vi "MSScript_Format_UpdDO.vi"(9 "ValueArray":string[](array[string]), 10 "TagArray":string[](array[string]), 11 "MSScript.lvclass":refnum<class "MSScript.lvclass">) -> (0 "ValueErrorArray":bool[](array[boolean]), 1 "TagErrorArray":bool[](array[boolean]), 2 "ParamErrorArray":bool[](array[boolean]), 3 "Data":variant, 4 "#ofParamError":bool)   [LabVIEW 2018, in "MSScript.lvclass"]
uses:
  MSScript.lvclass
  Ctl/MSEditorParam updDO.ctl
  MSScript_Transform_UIntArray.vi
  MSScript_Transform_BooleanArray.vi
panel:
  in  "ParamValueOutput":T1={"func"=[1, 2, 0, 0], "val"=[FALSE, FALSE, FALSE, FALSE]}
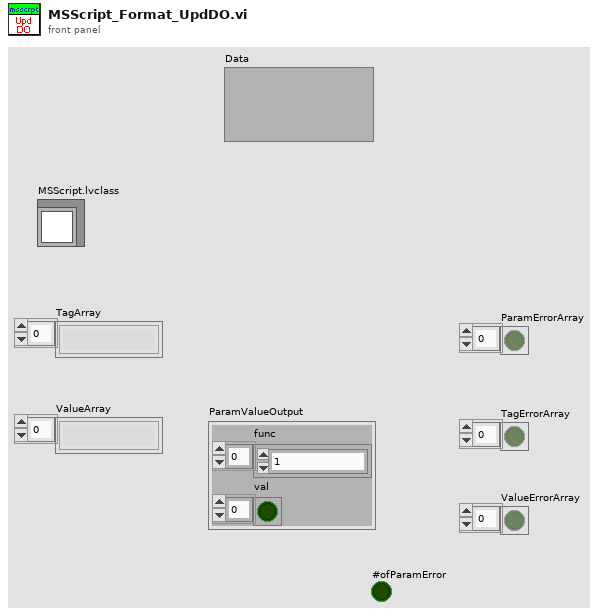
[diagram p1: front panel]
types:
  T1 = typedef "MSEditorParam updDO.ctl" = cluster{"func":u32[], "val":bool[]}
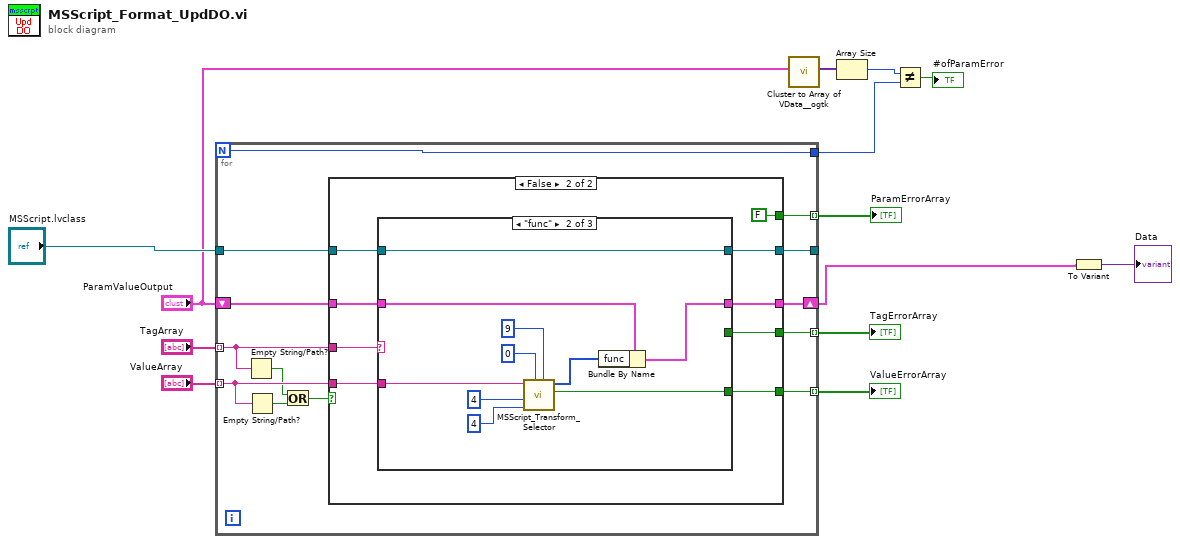
[diagram p0: block diagram]
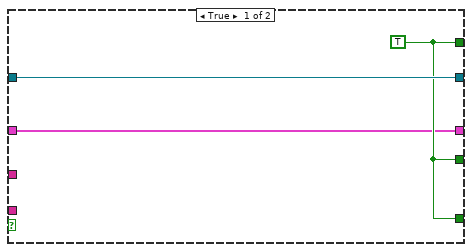
[diagram p2: hidden frame]
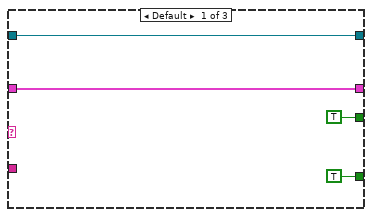
[diagram p3: hidden frame]
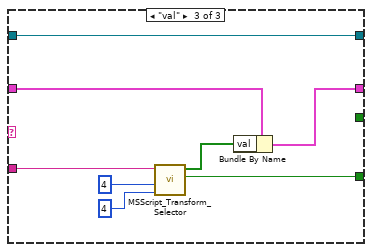
[diagram p4: hidden frame]
diagram:
  n1 = for {
    N -> [w14]
    tunnel: "TagArray" -> [w22] mode=indexing
    tunnel: "ValueArray" -> [w21] mode=indexing
    tunnel: [w26] -> w11 mode=indexing
    tunnel: "MSScript.lvclass" -> [w25]
    tunnel: [w24] -> w10 mode=indexing
    tunnel: [w23] -> _
    tunnel: [w17] -> w9 mode=indexing
    shift-right: [w15] -> w2
    shift-left: "ParamValueOutput" -> [w16]
    tunnel: [w14] -> w3
    n2 = Empty String/Path?(string/path=w22) -> (empty?=w19:bool)
    n3 = Empty String/Path?(string/path=w21) -> (empty?=w20:bool)
    n4 = Or(x=w19, y=w20) -> (x .or. y?=w18:bool)
    n5 = case shown="False" w18 {
      tunnel: [w28 w32] -> w26
      tunnel: w25 -> [w29 w37]
      tunnel: [w28 w33] -> w24
      tunnel: [w29 w30] -> w23
      tunnel: w22 -> [_ w35]
      tunnel: w21 -> [_ w34]
      tunnel: [w28 FALSE] -> w17
      tunnel: w16 -> [w27 w36]
      tunnel: [w27 w31] -> w15
      frame True {
        w28 = TRUE
      }
      frame False {
        n6 = case shown="\"func\"" w35 {
          tunnel: [TRUE _ _] -> w32
          tunnel: w37 -> [w40 w50 w58]
          tunnel: w34 -> [_ w51 w59]
          tunnel: [TRUE ("Value Error?") w52 w60] -> w33
          tunnel: [w40 w50 w58] -> w30
          tunnel: w36 -> [w39 w48 w56]
          tunnel: [w39 w47 w55] -> w31
          frame Default {
          }
          frame "func" {
            n7 = call-poly "MSScript_Transform_Selector.vi"("upper limit (18446744073709551615)"=u64 9 ("upper limit"), "lower limit (0)"=u64 0 ("lower limit"), "MinSize"=u8 4, "MaxSize"=u8 4, "Check_Str"=w51) -> ("Value Error?"=w52:bool, "Value Output"=w49:u64[])  [unwired: 4 in, 1 out]
            n8 = Bundle By Name(cluster=w48, "func"=w49) -> (w47:T1)
          }
          frame "val" {
            n9 = call-poly "MSScript_Transform_Selector.vi"("MinSize"=u8 4, "MaxSize"=u8 4, "Check_Str"=w59) -> ("Value Error?"=w60:bool, "Value Output"=w57:bool[])  [unwired: 7 in]
            n10 = Bundle By Name(cluster=w56, "val"=w57) -> (w55:T1)
          }
        }
      }
    }
  }
  "TagErrorArray" <- w11
  "ValueErrorArray" <- w10
  "ParamErrorArray" <- w9
  n11 = call <userlib>:"Cluster to Array of VData__ogtk.vi"("Cluster"="ParamValueOutput") -> ("Array of VData"=w7:variant[])  [unwired: 9 in, 1 out]
  n12 = Array Size(array=w7) -> (size(s)=w6:i32)
  n13 = Not Equal?(x=w6, y=w3) -> (x != y?=→"#ofParamError":bool)
  n14 = To Variant(anything=w2) -> (Variant=→"Data":variant)
